vi "Generate CtrlLabel-IOName config file.vi"() -> ()   [LabVIEW 2017]
uses:
  <vilib>/TELLC/CtrlRef/TD UI Control Label-Alias-IOName--cluster.ctl
  <vilib>/TELLC/CtrlRef/TD UI Control Label-IONames--cluster.ctl
panel:
  in  "MainUIPathname":path
  in  "ConfigFile":path=path "C:/Projects/Ichor/AVC2/Documents/ConfigFiles/CtrlLabel-IOName Config.ini"
  out "error out":errorcluster
  out "Size":i32
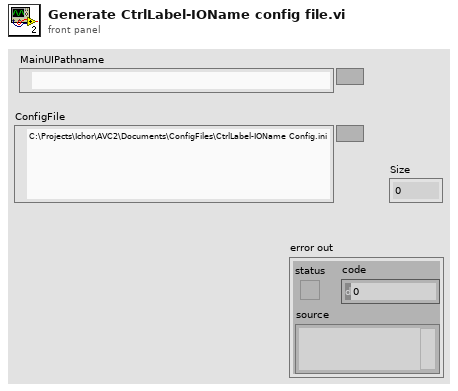
[diagram p1: front panel]
types:
  T1 = typedef "TD UI Control Label-IONames--cluster.ctl" = cluster{"Controls":T2[]}
  T2 = typedef "TD UI Control Label-Alias-IOName--cluster.ctl" = cluster{"Label":string, "Alias":string, "IOName":string}
  T3 = typedef "TD Pathnames--cluster.ctl" = cluster{"RunTimeSys?":bool, "AppFolder":path, "ExecutablePath":path, "ConfigFolder":path, "DataLogFolder":path, "SystemLogFolder":path, "SeqFolder":path, "MainStartupPathname":path, "MainUIPathname":path, "SystemEventsFile":path, "SeqEventsFile":path, "Config SettingsFile":path, "DAQ IOConfigFile":path, "SystemSimulation":bool}
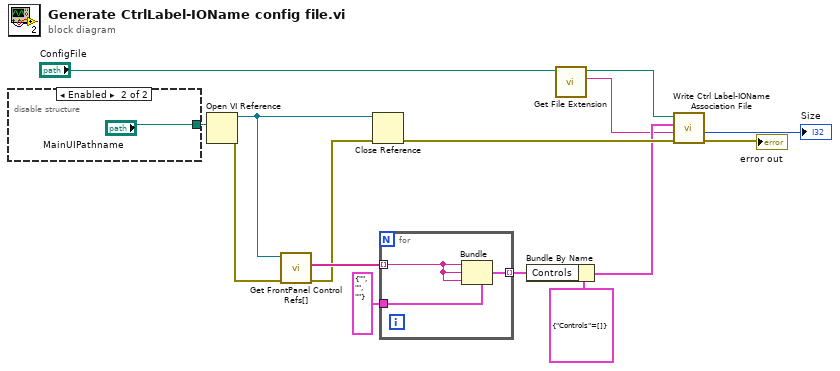
[diagram p0: block diagram]
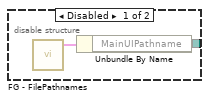
[diagram p2: hidden frame]
diagram:
  n1 = disable-structure shown="Enabled" {
    disable-tunnel: [w17 "MainUIPathname"] -> w15
    frame Disabled {
      n2 = call "FG - FilePathnames.vi"() -> ("FilePaths out"=w16:T3)  [unwired: 4 in, 1 out]
      n3 = Unbundle By Name(w16) -> ("MainUIPathname"=w17:path)
    }
    frame Enabled {
    }
  }
  n4 = Open VI Reference(vi path=w15) -> (vi reference=w14:refnum<vi>, error out=w11:errorcluster)  [unwired: 5 in]
  n5 = call <vilib>:"Get FrontPanel Control Refs[].vi"("error in"=w11, "VI (Caller)"=w14) -> ("error out"=w8:errorcluster, "Labels[]"=w13:string[])  [unwired: 7 in, 1 out]
  n6 = Close Reference(reference=w14, error in (no error)=w8) -> (error out=w7:errorcluster)
  n7 = for {
    tunnel: w13 -> [w19] mode=indexing
    tunnel: T2 {"Label"="", "Alias"="", "IOName"=""} ("Label Associations") -> [w21]
    tunnel: [w20] -> w9 mode=indexing
    n8 = Bundle(cluster=w21, "Label"=w19, "Alias"=w19, "IOName"=w19) -> (w20:T2)
  }
  n9 = Bundle By Name(cluster=T1 {"Controls"=[]} ("UI Control Label Associations"), "Controls"=w9) -> (w6:T1)
  n10 = call <vilib>:"Get File Extension.vi"("file"="ConfigFile") -> ("lowercase file extension"=w1:string, "dup file"=w2:path)  [unwired: 6 in, 3 out]
  n11 = call <vilib>:"Write Ctrl Label-IOName Association File.vi"("error in (no error)"=w7, "file extension"=w1, "UI Control Label Associations"=w6, "ConfigFile"=w2) -> ("error out"=→"error out":errorcluster, "Size"=→"Size":i32)  [unwired: 6 in]
